vi "Slice Row (DVR).vi"(6 "Fake Point (0)":dbl, 8 "error in (no error)":errorcluster, 9 "Row":i32, 10 "Page":i32, 11 "Data Value Reference in":refnum<data-value>) -> (0 "error out":errorcluster, 2 "X-array":dbl[](array[numeric]), 3 "2D Array":dbl[][](array[numeric]))   [LabVIEW 2016, in "Retrieve and Visualize.lvclass"]
uses:
  Retrieve and Visualize.lvclass
  <userlib>/LevyLab/XY Utilities/Typedefs/Interpolation Configuration--cluster.ctl
  <userlib>/LevyLab/XY Utilities/subVIs/Get X and Y (single).vi
  <userlib>/LevyLab/XY Utilities/subVIs/Interpolate (multiple).vi
  <userlib>/LevyLab/XY Utilities/xy_utilities.lvlib
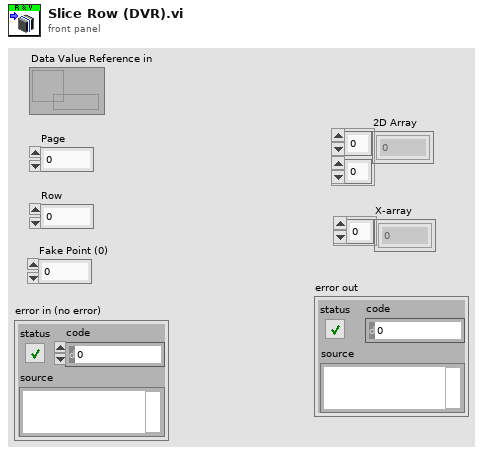
[diagram p1: front panel]
types:
  T1 = typedef "xy_utilities.lvlib/Interpolation Configuration--cluster.ctl" = cluster{"X Low":dbl, "X High":dbl, "X Step":dbl, "Fake Point":dbl}
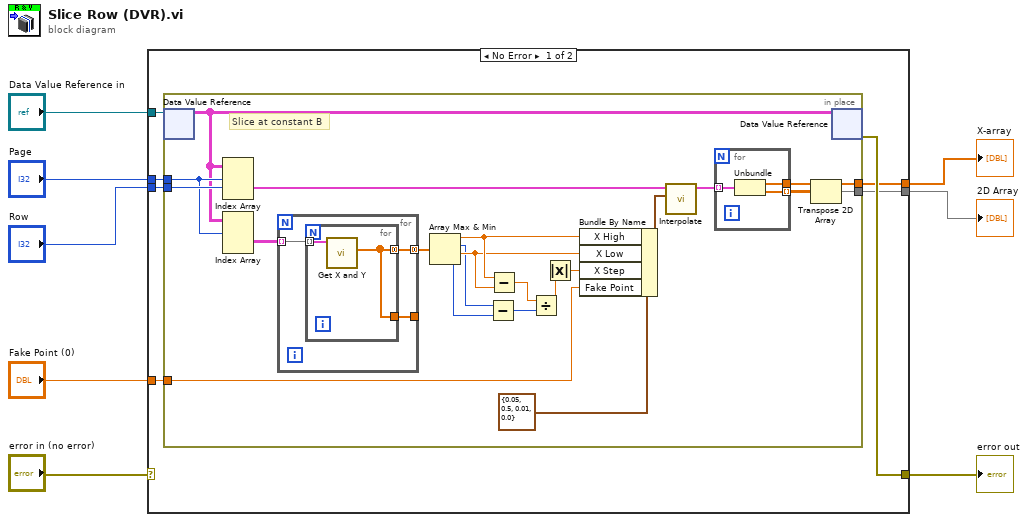
[diagram p0: block diagram]
diagram:
  n1 = case shown="No Error" "error in (no error)" {
    selector: "error in (no error)" -> [_ w45]
    tunnel: "Row" -> [w15 _]
    tunnel: "Page" -> [w14 _]
    tunnel: "Fake Point (0)" -> [w13 _]
    tunnel: "Data Value Reference in" -> [w12 _]
    tunnel: [w11 w45] -> w4
    tunnel: [w10 _] -> w2
    tunnel: [w9 _] -> w1
    frame No Error {
      n2 = in-place {
        in-place-border: [w31] -> w9
        in-place-border: [w33] -> w10
        in-place-border: w14 -> [w30]
        in-place-border: w15 -> [w32]
        in-place-border: w13 -> [w23]
        # "Slice at constant B"
        n3 = in-place-dvr #1(w12) -> (w22:cluster{dbl[], dbl[]}[][][])  [unwired: 1 out]
        n4 = Index Array(array=w22, index (dim 0)=w30, index (dim 1)=w32) -> (element=w34:cluster{dbl[], dbl[]}[])  [unwired: 1 in]
        n5 = Index Array(array=w22, index (dim 0)=w30) -> (element=w29:cluster{dbl[], dbl[]}[][])  [unwired: 2 in]
        n6 = for {
          tunnel: w29 -> [w39] mode=indexing
          tunnel: [w38] -> w28 mode=concatenating
          tunnel: [w37] -> _
          n7 = for {
            tunnel: w39 -> [w41] mode=indexing
            tunnel: [w40] -> w38 mode=concatenating
            tunnel: [w40] -> w37
            n8 = call-poly <userlib>:"Get X and Y.vi"("XY-data"=w41) -> ("X-array"=w40:dbl[])  [unwired: 7 in, 3 out]
          }
        }
        n9 = Array Max & Min(array=w28) -> (max value=w25:dbl, max index (indices)=w21:i32, min value=w24:dbl, min index (indices)=w20:i32)
        n10 = Subtract(x=w21, y=w20) -> (x-y=w19:i32)
        n11 = Subtract(x=w25, y=w24) -> (x-y=w18:dbl)
        n12 = Divide(x=w18, y=w19) -> (x/y=w16:dbl)
        n13 = Absolute Value(x=w16) -> (abs(x)=w17:dbl)
        n14 = Bundle By Name(cluster=T1 {"X Low"=0.05, "X High"=0.5, "X Step"=0.01, "Fake Point"=0.0} ("Configure"), "X High"=w25, "X Low"=w24, "X Step"=w17, "Fake Point"=w23) -> (w26:T1)
        n15 = call-poly <userlib>:"Interpolate.vi"("Configure"=w26, "XY-data"=w34) -> ("Interpolated XY-data out"=w36:cluster{"X-array":dbl[], "Y-array":dbl[]}[])  [unwired: 8 in, 1 out]
        n16 = for {
          tunnel: [w44] -> w33
          tunnel: [w43] -> w35 mode=indexing
          tunnel: w36 -> [w42] mode=indexing
          n17 = Unbundle(w42) -> ("X-array"=w44:dbl[], "Y-array"=w43:dbl[])
        }
        n18 = Transpose 2D Array(2D array=w35) -> (transposed array=w31:dbl[][])
        n19 = in-place-dvr #1(w22) -> (w11:errorcluster)  [unwired: 1 out]
      }
    }
    frame Error {
    }
  }
  "X-array" <- w2
  "2D Array" <- w1
  "error out" <- w4
